vi "Speech-OpenVoiceObjects.vi"(8 "error in (no error)":errorcluster) -> (0 "error out":errorcluster, 1 "Voice Names":string[](array[string]), 2 "AudioDevices":string[](array[string]), 3 "speech_voice_refs":T1)   [LabVIEW 8.6]
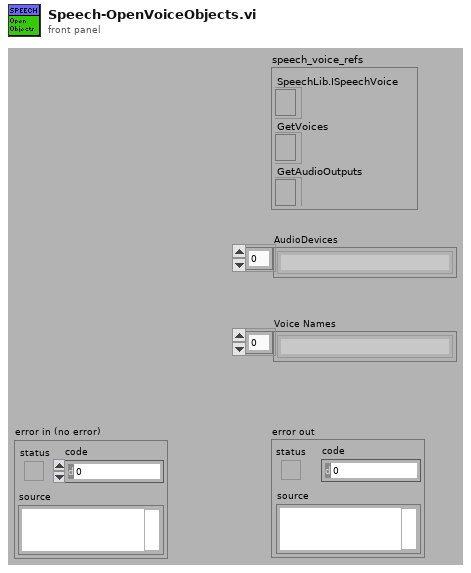
[diagram p1: front panel]
types:
  T1 = cluster{"SpeechLib.ISpeechVoice":refnum<k7>, "GetVoices":refnum<k7>, "GetAudioOutputs":refnum<k7>}
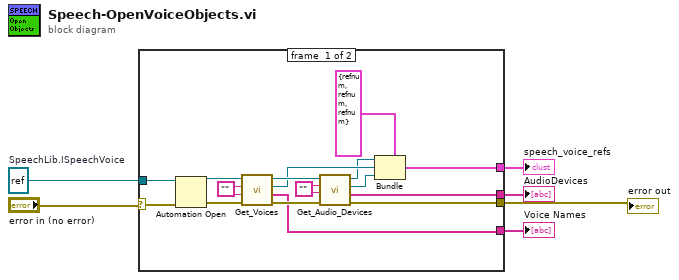
[diagram p0: block diagram]
diagram:
  w5 = refnum<k7> refnum  # SpeechLib.ISpeechVoice
  n1 = case shown="No Error" "error in (no error)" {
    selector: "error in (no error)" -> [w19 _]
    tunnel: w5 -> [w22 _]
    tunnel: [w11 _] -> w2
    tunnel: [w10 _] -> w3
    tunnel: [w9 _] -> w1
    tunnel: [w7 _] -> w4
    frame #0 {
      w8 = ""
      w16 = ""
      n2 = Automation Open(error in (no error)=w19, Automation Refnum=w22) -> (Automation Refnum=w21:refnum<k7>, error out=w20:errorcluster)  [unwired: 2 in]
      n3 = call "Get_Voices.vi"("error out"=w20, "OptionalAttributes"=w16, "RequiredAttributes"=w16, "SpeechLib.ISpeechVoice (In)"=w21) -> ("error out"=w18:errorcluster, "Voice Names"=w9:string[], "GetVoices (Out)"=w13:refnum<k7>, "SpeechLib.ISpeechVoice (Out)"=w17:refnum<k7>)
      n4 = call "Get_Audio_Devices.vi"("error in"=w18, "OptionalAttributes"=w8, "RequiredAttributes"=w8, "SpeechLib.ISpeechVoice (In)"=w17) -> ("error out"=w11:errorcluster, "AudioDevices"=w10:string[], "GetAudioOutputs"=w14:refnum<k7>, "SpeechLib.ISpeechVoice (Out)"=w12:refnum<k7>)
      n5 = Bundle(cluster=T1 {"SpeechLib.ISpeechVoice"=refnum, "GetVoices"=refnum, "GetAudioOutputs"=refnum} ("speech object references"), "SpeechLib.ISpeechVoice"=w12, "GetVoices"=w13, "GetAudioOutputs"=w14) -> (w7:T1)
    }
    frame #1 {
    }
  }
  "speech_voice_refs" <- w4
  "AudioDevices" <- w3
  "error out" <- w2
  "Voice Names" <- w1
